vi "SimpleCurrentRead.vi"(8 "error in (no error)":errorcluster, 9 "Current Setting":dbl, 10 "Function (0: Volts)":u16=1, 11 "Keithley In":refnum<visa-resource-name>) -> (0 "error out":errorcluster, 2 "Measured Current":dbl, 3 "Keithley Out":refnum<visa-resource-name>)   [LabVIEW 2013]
uses:
  <instrlib>/Keithley 24XX/Public/Data/Read (Single Point).vi
  <instrlib>/Keithley 24XX/Keithley 24XX.lvlib
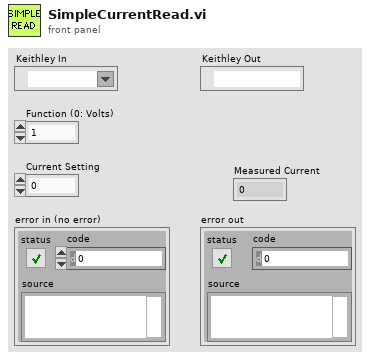
[diagram p1: front panel]
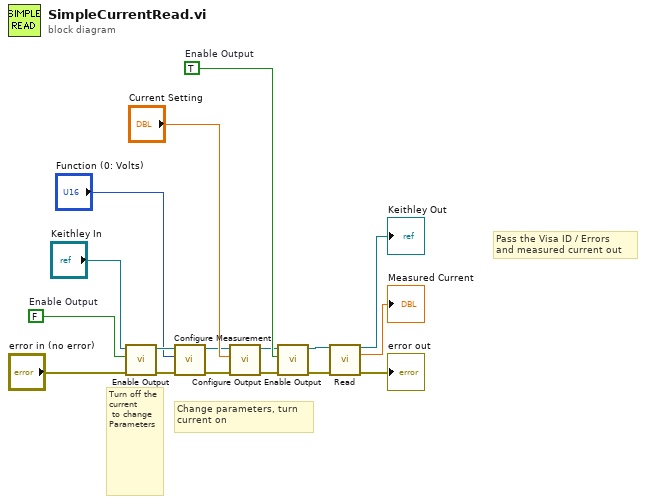
[diagram p0: block diagram]
diagram:
  w14 = TRUE  # Enable Output
  w6 = FALSE  # Enable Output
  # "Pass the Visa ID / Errors \nand measured current out"
  # "Change parameters, turn current on"
  # "Turn off the current\n to change Parameters"
  n1 = call <instrlib>:"Enable Output.vi"("error in (no error)"="error in (no error)", "Enable Output (T: Enable)"=w6, "VISA resource name"="Keithley In") -> ("error out"=w2:errorcluster, "VISA resource name out"=w3:refnum<visa-resource-name>)  [unwired: 7 in]
  n2 = call <instrlib>:"Configure Measurement.vi"("error in (no error)"=w2, "Function (0: Volts)"="Function (0: Volts)", "VISA resource name"=w3) -> ("error out"=w15:errorcluster, "VISA resource name out"=w16:refnum<visa-resource-name>)  [unwired: 7 in]
  n3 = call <instrlib>:"Configure Output.vi"("error in (no error)"=w15, "Output Level (0)"="Current Setting", "VISA resource name"=w16) -> ("error out"=w13:errorcluster, "VISA resource name out"=w12:refnum<visa-resource-name>)  [unwired: 7 in]
  n4 = call <instrlib>:"Enable Output.vi"("error in (no error)"=w13, "Enable Output (T: Enable)"=w14, "VISA resource name"=w12) -> ("error out"=w10:errorcluster, "VISA resource name out"=w11:refnum<visa-resource-name>)  [unwired: 7 in]
  n5 = call-poly <instrlib>:"Read.vi"("VISA resource name"=w11, "error in (no error)"=w10) -> ("VISA resource name out"=→"Keithley Out":refnum<visa-resource-name>, "Current"=→"Measured Current":sgl, "error out"=→"error out":errorcluster)  [unwired: 7 in, 4 out]
